vi "Light a Scene.vi"() -> ()   [LabVIEW 2023]
doc: "This VI demonstrates how to create a more complex hierarchy of objects and add light to the scene. It also demonstrates how to control the light and programmatically change position and light."
uses:
  <vilib>/picture/3D Picture Control/Object/Create Object (name).vi
  <vilib>/picture/3D Picture Control/Object/Create Object (drawable).vi
  <vilib>/picture/3D Picture Control/Helpers/Apply Texture (reference).vi
  <vilib>/picture/3D Picture Control/Object/Add Object (no reference).vi
  <vilib>/picture/3D Picture Control/Helpers/Set Light (reference).vi
  <vilib>/picture/3D Picture Control/NI_3D Picture Control.lvlib
panel:
  in  "Fixed light height":sgl(slide)=500.0 scale=1.0..500.0
  in  "Frequency":dbl(knob)=-0.3148884514230843 scale=-1.0..1.0
  in  "Rotating Light":bool=TRUE
  in  "Fixed Light":bool=TRUE
  in  "Texture Mode":T1(ring)=enum."With Modulation"
  in  "Radius":dbl(slide)=14.545454545454545 scale=0.0..20.0
  in  "Rotating light height":sgl(slide)=5.3061223 scale=0.0..20.0
  in  "Stop":bool
  out "3D Picture":refnum<vi>(3d-picture)
  # "Overview: This VI demonstrates how to create a more complex hierarchy of objects and add light to the scene in a 3D Picture. \nRequirements: LabVIEW Full Development System\nInstructions: \n1. Run the VI.\n2. Observe the appearance of the image when the Rotating Light and Fixed Light are turned on and off.\n3. Observe the appearance of the image when the Rotating light height and Fixed light height are changed.\n4. Click Stop to stop the VI."
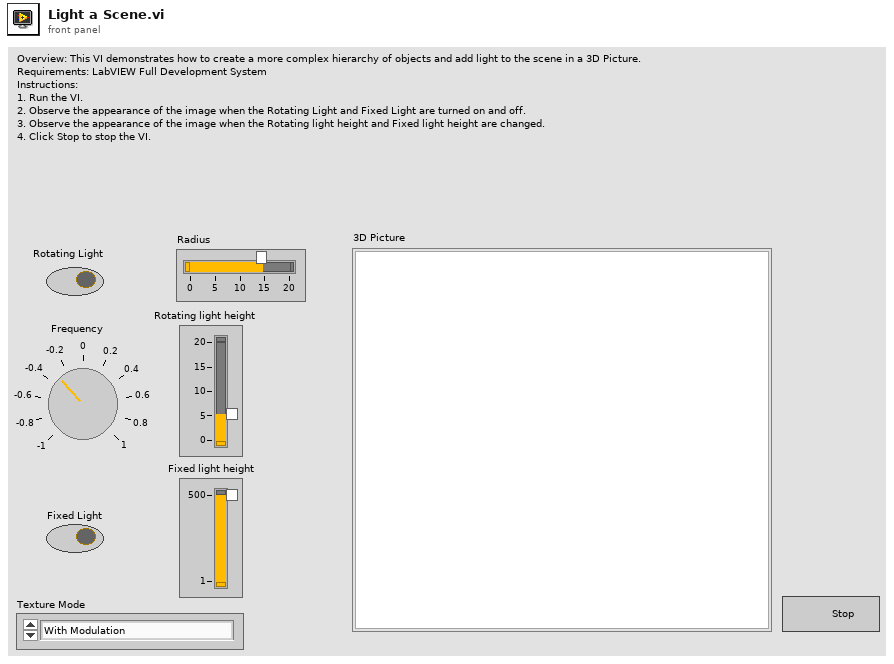
[diagram p1: front panel]
types:
  T1 = enum16{"As a Decal", "With Modulation", "With Blending", "As a replacement"}
  T2 = typedef "imagedata.ctl" = cluster{"image type":i32, "image depth":i32, "image":u8[], "mask":u8[], "colors":u32[], "Rectangle":cluster{"left":i16, "top":i16, "right":i16, "bottom":i16}}
  T3 = cluster{"x*y":dbl, "x*y":dbl, "Fixed light height":sgl}
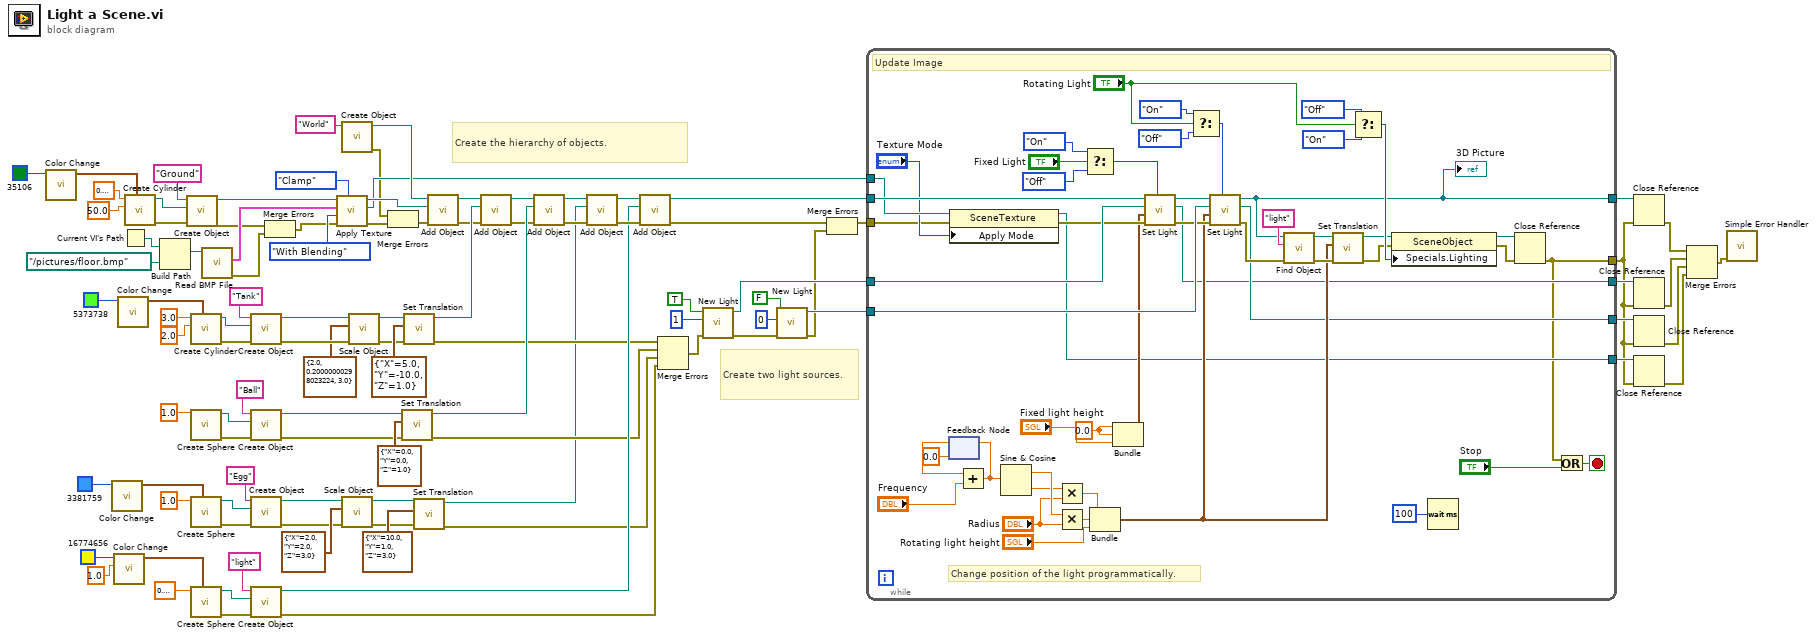
[diagram p0: block diagram]
diagram:
  # "Create two light sources."
  # "Create the hierarchy of objects."
  n1 = call <vilib>:"Color Change.vi"("Color"=u32 35106) -> ("RGBA"=w99:cluster{"R":sgl, "G":sgl, "B":sgl, "A":sgl})  [unwired: 10 in]
  n2 = call <vilib>:"Color Change.vi"("Color"=u32 3381759) -> ("RGBA"=w56:cluster{"R":sgl, "G":sgl, "B":sgl, "A":sgl})  [unwired: 10 in]
  n3 = call <vilib>:"Color Change.vi"("Alpha"=1.0, "Color"=u32 16774656) -> ("RGBA"=w83:cluster{"R":sgl, "G":sgl, "B":sgl, "A":sgl})  [unwired: 9 in]
  n4 = call <vilib>:"Color Change.vi"("Color"=u32 5373738) -> ("RGBA"=w59:cluster{"R":sgl, "G":sgl, "B":sgl, "A":sgl})  [unwired: 10 in]
  n5 = Current VI's Path() -> (path=w11:path)
  n6 = call <vilib>:"Create Cylinder.vi"("Color"=w99, "Radius"=sgl 50.0 ("Height"), "Height"=sgl 0.1) -> ("error out"=w46:errorcluster, "New Cylinder Refnum"=w100:refnum<vi>)  [unwired: 7 in]
  n7 = Build Path(base path=w11, name or relative path=path "../pictures/floor.bmp" ("path")) -> (appended path=w101:path)
  n8 = call-poly <vilib>:"Create Object.vi"("error in (no error)"=w46, "Geometry"=w100, "Name"="Ground") -> ("error out"=w45:errorcluster, "Scene:New Object"=w95:refnum<vi>)  [unwired: 7 in]
  n9 = call <vilib>:"Create Cylinder.vi"("Color"=w59, "Radius"=sgl 2.0, "Height"=sgl 3.0 ("Radius")) -> ("error out"=w38:errorcluster, "New Cylinder Refnum"=w65:refnum<vi>)  [unwired: 7 in]
  n10 = call <vilib>:"Create Sphere.vi"("Radius"=sgl 1.0) -> ("error out"=w37:errorcluster, "New Sphere Refnum"=w91:refnum<vi>)  [unwired: 9 in]
  n11 = call <vilib>:"Create Sphere.vi"("Color"=w56, "Radius"=sgl 1.0) -> ("error out"=w85:errorcluster, "New Sphere Refnum"=w86:refnum<vi>)  [unwired: 8 in]
  n12 = call <vilib>:"Create Sphere.vi"("Color"=w83, "Radius"=sgl 0.3) -> ("error out"=w39:errorcluster, "New Sphere Refnum"=w79:refnum<vi>)  [unwired: 8 in]
  n13 = call <vilib>:"Read BMP File.vi"("path to BMP file"=w101) -> ("error out"=w43:errorcluster, "image data"=w92:T2)  [unwired: 8 in, 1 out]
  n14 = call-poly <vilib>:"Create Object.vi"("error in (no error)"=w38, "Geometry"=w65, "Name"="Tank") -> ("error out"=w36:errorcluster, "Scene:New Object"=w50:refnum<vi>)  [unwired: 7 in]
  n15 = call-poly <vilib>:"Create Object.vi"("error in (no error)"=w37, "Geometry"=w91, "Name"="Ball") -> ("error out"=w33:errorcluster, "Scene:New Object"=w77:refnum<vi>)  [unwired: 7 in]
  n16 = call-poly <vilib>:"Create Object.vi"("error in (no error)"=w85, "Geometry"=w86, "Name"="Egg") -> ("error out"=w16:errorcluster, "Scene:New Object"=w17:refnum<vi>)  [unwired: 7 in]
  n17 = call-poly <vilib>:"Create Object.vi"("error in (no error)"=w39, "Geometry"=w79, "Name"="light") -> ("error out"=w24:errorcluster, "Scene:New Object"=w68:refnum<vi>)  [unwired: 7 in]
  n18 = Merge Errors(w45, w43) -> (w44:errorcluster)
  n19 = call-poly <vilib>:"Apply Texture.vi"("Horizontal Wrap Mode"=enum16{"Clamp", "Repeat"}."Clamp", "error in (no error)"=w44, "Apply Mode"=T1."With Blending", "Image Data"=w92, "Scene Object In"=w95) -> ("error out"=w41:errorcluster, "Texture Refnum"=w47:refnum<vi>, "Scene Object Out"=w94:refnum<vi>)  [unwired: 4 in]
  n20 = call-poly <vilib>:"Create Object.vi"("Name"="World") -> ("error out"=w40:errorcluster, "Scene:New Object"=w93:refnum<vi>)  [unwired: 9 in]
  n21 = call <vilib>:"Scale Object.vi"("error in (no error)"=w16, "Scale"=cluster{"X":sgl, "Y":sgl, "Z":sgl} {"X"=2.0, "Y"=2.0, "Z"=3.0} ("Translation"), "Scene.Object In"=w17) -> ("error out"=w15:errorcluster, "Scene.Object Out"=w13:refnum<vi>)  [unwired: 7 in]
  n22 = call <vilib>:"Scale Object.vi"("error in (no error)"=w36, "Scale"=cluster{"X":sgl, "Y":sgl, "Z":sgl} {"X"=2.0, "Y"=0.2, "Z"=3.0} ("Translation"), "Scene.Object In"=w50) -> ("error out"=w35:errorcluster, "Scene.Object Out"=w49:refnum<vi>)  [unwired: 7 in]
  n23 = Merge Errors(w40, w41) -> (w42:errorcluster)
  n24 = call <vilib>:"Set Translation.vi"("error in (no error)"=w33, "Translation"=cluster{"X":sgl, "Y":sgl, "Z":sgl} {"X"=0.0, "Y"=0.0, "Z"=1.0}, "Scene Object"=w77) -> ("error out"=w25:errorcluster, "Translated Object"=w76:refnum<vi>)  [unwired: 7 in]
  n25 = call <vilib>:"Set Translation.vi"("error in (no error)"=w35, "Translation"=cluster{"X":sgl, "Y":sgl, "Z":sgl} {"X"=5.0, "Y"=-10.0, "Z"=1.0}, "Scene Object"=w49) -> ("error out"=w26:errorcluster, "Translated Object"=w48:refnum<vi>)  [unwired: 7 in]
  n26 = call <vilib>:"Set Translation.vi"("error in (no error)"=w15, "Translation"=cluster{"X":sgl, "Y":sgl, "Z":sgl} {"X"=10.0, "Y"=1.0, "Z"=3.0}, "Scene Object"=w13) -> ("error out"=w14:errorcluster, "Translated Object"=w12:refnum<vi>)  [unwired: 7 in]
  n27 = call-poly <vilib>:"Add Object.vi"("error in (no error)"=w42, "New Object In"=w94, "Scene Object In"=w93) -> ("error out"=w31:errorcluster, "Scene Object Out"=w63:refnum<vi>)  [unwired: 7 in]
  n28 = call-poly <vilib>:"Add Object.vi"("error in (no error)"=w31, "New Object In"=w48, "Scene Object In"=w63) -> ("error out"=w30:errorcluster, "Scene Object Out"=w64:refnum<vi>)  [unwired: 7 in]
  n29 = call-poly <vilib>:"Add Object.vi"("error in (no error)"=w30, "New Object In"=w76, "Scene Object In"=w64) -> ("error out"=w29:errorcluster, "Scene Object Out"=w75:refnum<vi>)  [unwired: 7 in]
  n30 = call-poly <vilib>:"Add Object.vi"("error in (no error)"=w29, "New Object In"=w12, "Scene Object In"=w75) -> ("error out"=w69:errorcluster, "Scene Object Out"=w74:refnum<vi>)  [unwired: 7 in]
  n31 = call-poly <vilib>:"Add Object.vi"("error in (no error)"=w69, "New Object In"=w68, "Scene Object In"=w74) -> ("error out"=w23:errorcluster, "Scene Object Out"=w73:refnum<vi>)  [unwired: 7 in]
  n32 = Merge Errors(w26, w25, w14, w24) -> (w21:errorcluster)
  n33 = call <vilib>:"New Light.vi"("error in (no error)"=w21, "Light Number"=1, "At Infinity"=TRUE) -> ("error out"=w20:errorcluster, "New Light Refnum"=w88:refnum<vi>)  [unwired: 7 in]
  n34 = call <vilib>:"New Light.vi"("error in (no error)"=w20, "Light Number"=0, "At Infinity"=FALSE) -> ("error out"=w19:errorcluster, "New Light Refnum"=w55:refnum<vi>)  [unwired: 7 in]
  n35 = Merge Errors(w23, w19) -> (w22:errorcluster)
  n36 = while {
    tunnel: w73 -> [w139]
    tunnel: w47 -> [w138]
    tunnel: w22 -> [w119]
    tunnel: [w103] -> w2
    tunnel: [w107] -> w4
    tunnel: [w106] -> w3
    tunnel: w88 -> [w140]
    tunnel: [w108] -> w10
    tunnel: w55 -> [w135]
    tunnel: [w109] -> w9
    stop <- w114 stop-if-true
    w121 = 0.0 ("x*y")
    # "Change position of the light programmatically."
    # "Update Image"
    n37 = feedback #1(0.0) -> (w123:dbl)
    n38 = property class="SceneTexture"(reference=w138, error in=w119, "Apply Mode"="Texture Mode") -> (reference out=w106:refnum<vi>, error out=w118:errorcluster)
    n39 = Add(x=w123, y="Frequency") -> (x+y=w124:dbl)
    n40 = feedback-in #1(w124) -> ()
    n41 = Sine & Cosine(0:w124) -> (1:w149:dbl, 2:w148:dbl)
    n42 = Multiply(x=w148, y="Radius") -> (x*y=w141:dbl)
    n43 = Multiply(x=w149, y="Radius") -> (x*y=w146:dbl)
    n44 = Select(t=enum16{"Inherit Value", "Off", "On"}."On" ("Light State 2"), s="Fixed Light", f=enum16{"Inherit Value", "Off", "On"}."Off" ("Light State 2")) -> (s? t:f=w128:enum16{"Inherit Value", "Off", "On"})
    n45 = Bundle(w141, w146, "Rotating light height"="Rotating light height") -> (w111:cluster{dbl, dbl, "Rotating light height":sgl})  [unwired: 1 in]
    n46 = Bundle("x*y"=w121, "x*y"=w121, "Fixed light height"="Fixed light height") -> (w112:T3)  [unwired: 1 in]
    n47 = call-poly <vilib>:"Set Light.vi"("Light State"=w128, "error in (no error)"=w118, "Position"=w112, "Light Refnum In"=w140, "Scene Object In"=w139) -> ("error out"=w134:errorcluster, "Light Refnum Out"=w108:refnum<vi>, "Scene Object Out"=w136:refnum<vi>)  [unwired: 4 in]
    n48 = Select(t=enum16{"Inherit Value", "Off", "On"}."On" ("Light State 2"), s="Rotating Light", f=enum16{"Inherit Value", "Off", "On"}."Off" ("Light State 2")) -> (s? t:f=w133:enum16{"Inherit Value", "Off", "On"})
    n49 = call-poly <vilib>:"Set Light.vi"("Light State"=w133, "error in (no error)"=w134, "Position"=w111, "Light Refnum In"=w135, "Scene Object In"=w136) -> ("error out"=w110:errorcluster, "Light Refnum Out"=w109:refnum<vi>, "Scene Object Out"=w107:refnum<vi>)  [unwired: 4 in]
    "3D Picture" <- w107
    n50 = call <vilib>:"Find Object.vi"("error in (no error)"=w110, "Object Name"="light", "Scene Refnum"=w107) -> ("error out"=w142:errorcluster, "Object Refnum"=w116:refnum<vi>)  [unwired: 7 in]
    n51 = call <vilib>:"Set Translation.vi"("error in (no error)"=w142, "Translation"=w111, "Scene Object"=w116) -> ("error out"=w117:errorcluster, "Translated Object"=w115:refnum<vi>)  [unwired: 7 in]
    n52 = Select(t=enum16{"Inherit Value", "Off", "On"}."Off" ("Specials:Lighting"), s="Rotating Light", f=enum16{"Inherit Value", "Off", "On"}."On" ("Specials:Lighting")) -> (s? t:f=w127:enum16{"Inherit Value", "Off", "On"})
    n53 = property class="SceneObject"(reference=w115, error in=w117, "Specials.Lighting"=w127) -> (reference out=w105:refnum<vi>, error out=w104:errorcluster)
    n54 = Wait (ms)(milliseconds to wait=u32 100 ("millisecond multiple")) -> ()  [unwired: 1 out]
    n55 = Close Reference(reference=w105, error in (no error)=w104) -> (error out=w103:errorcluster)
    n56 = Or(x=w103, y="Stop") -> (x .or. y?=w114:bool)
  }
  n57 = Close Reference(reference=w4, error in (no error)=w2) -> (error out=w6:errorcluster)
  n58 = Close Reference(reference=w10, error in (no error)=w2) -> (error out=w7:errorcluster)
  n59 = Close Reference(reference=w9, error in (no error)=w2) -> (error out=w8:errorcluster)
  n60 = Close Reference(reference=w3, error in (no error)=w2) -> (error out=w1:errorcluster)
  n61 = Merge Errors(w6, w7, w8, w1) -> (w5:errorcluster)
  n62 = call <vilib>:"Simple Error Handler.vi"("error in (no error)"=w5) -> ()  [unwired: 4 in, 5 out]
